vi "Read sort_.vi"(8 "error in":errorcluster, 11 "user tag bus module editor node in":refnum<class "fixed channel tag bus module editor node.lvclass">) -> (0 "error out":errorcluster, 2 "sort?":bool, 3 "user tag bus module editor node out":refnum<class "fixed channel tag bus module editor node.lvclass">)   [LabVIEW 2013, in "fixed channel tag bus module editor node.lvclass"]
uses:
  fixed channel tag bus module editor node.lvclass
  fixed channel tag bus module editor node.lvclass/fixed channel tag bus module editor node.ctl
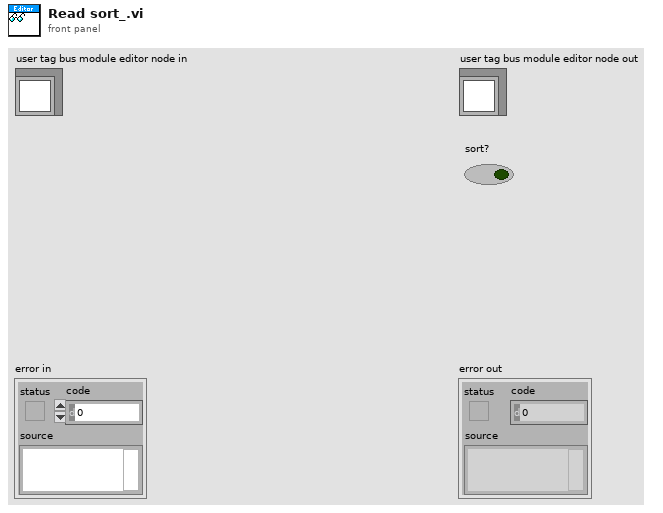
[diagram p1: front panel]
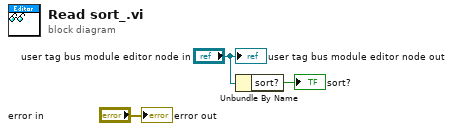
[diagram p0: block diagram]
diagram:
  n1 = Unbundle By Name("user tag bus module editor node in") -> ("sort?"=→"sort?":bool)
  "error out" <- "error in"
  "user tag bus module editor node out" <- "user tag bus module editor node in"
